vi "Create.vi"(10 "ID":string) -> (3 "Module Identity out":refnum<class "Module Identity.lvclass">)   [LabVIEW 2020, in "Volatus.lvlib" / "Module Identity.lvclass"]
uses:
  Module Identity.lvclass
  Module Identity.lvclass/Module Identity.ctl
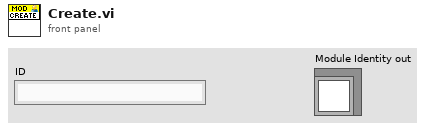
[diagram p1: front panel]
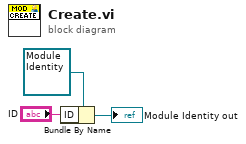
[diagram p0: block diagram]
diagram:
  n1 = Bundle By Name(cluster=refnum<class "Module Identity.lvclass"> refnum ("Module Identity in"), "ID"="ID") -> (→"Module Identity out":refnum<class "Module Identity.lvclass">)
